vi "I-O Test.vi"() -> ()   [LabVIEW 2016]
uses:
  Classes/Controller/I-O/I-O.lvclass
  Classes/Controller/Controller.lvclass
panel:
  in  "secondary valve":bool
  in  "primary valve":bool
  out "Compression":bool=TRUE
  in  "Region Index":i32=1
  in  "Position Index":i32
  in  "Write":bool
  out "Read":bool
  in  "Stop":bool
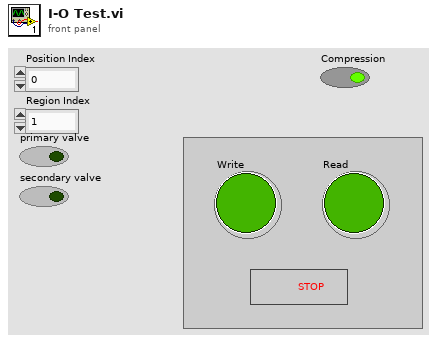
[diagram p1: front panel]
types:
  T1 = typedef "Controller.lvclass/Controllers.ctl" = cluster{"I-O.lvclass":refnum<class "I-O.lvclass">, "Motion.lvclass":refnum<class "Motion.lvclass">, "Dispenser.lvclass":refnum<class "Dispenser.lvclass">}
  T2 = typedef "I-O.lvclass/Pin Map.ctl" = cluster{"Region Valves":i32[], "Extra Valves":dbl[][], "Tool Primary Valve":i32, "Tool Secondary Valve":i32, "Region Sensors":i32[], "Extra Sensors":dbl[][], "Tool Primary Sensor":dbl, "Tool Secondary Sensor":dbl, "Compression Sensor":dbl, "5V":i32}
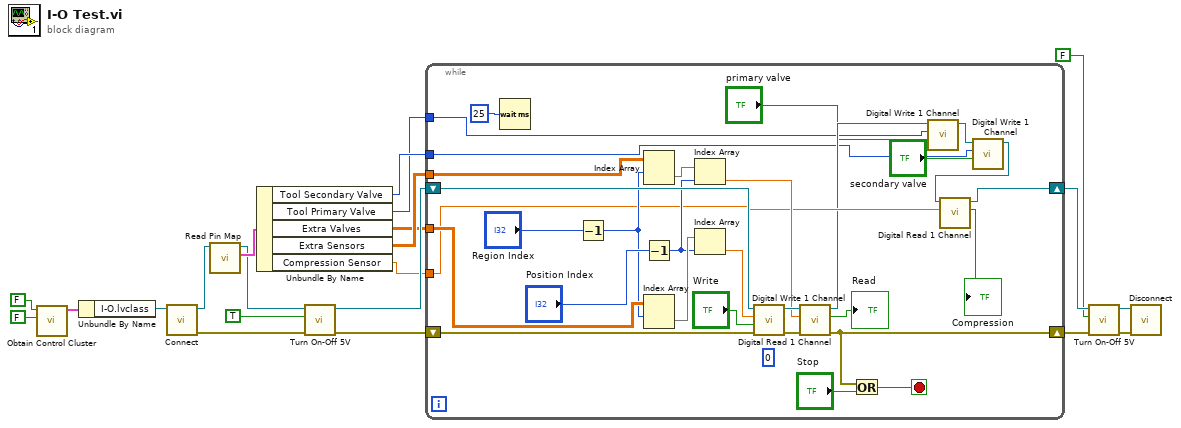
[diagram p0: block diagram]
diagram:
  n1 = call "Obtain Control Cluster.vi"("Dispense"=FALSE, "Motion"=FALSE) -> ("Control Out"=w5:T1)  [unwired: 9 in]
  n2 = Unbundle By Name(w5) -> ("I-O.lvclass"=w4:refnum<class "I-O.lvclass">)
  n3 = call-dynamic "Connect.vi"("Controller in"=w4) -> ("error out"=w12:errorcluster, "Controller out"=w14:refnum<class "I-O.lvclass">)  [unwired: 9 in]
  n4 = call-dynamic "Read Pin Map.vi"("I-O in"=w14) -> ("Pin Map"=w16:T2, "I-O out"=w15:refnum<class "I-O.lvclass">)  [unwired: 8 in, 1 out]
  n5 = Unbundle By Name(w16) -> ("Tool Secondary Valve"=w2:i32, "Tool Primary Valve"=w1:i32, "Extra Valves"=w8:dbl[][], "Extra Sensors"=w13:dbl[][], "Compression Sensor"=w3:dbl)
  n6 = call-dynamic "Turn On-Off 5V.vi"("error in (no error)"=w12, "Value"=TRUE, "I-O in"=w15) -> ("error out"=w11:errorcluster, "I-O out"=w21:refnum<class "I-O.lvclass">)  [unwired: 7 in]
  n7 = while {
    shift-right: [w29] -> w18
    shift-left: w21 -> [w50]
    tunnel: w13 -> [w37]
    shift-right: [w44] -> w10
    shift-left: w11 -> [w46]
    tunnel: w8 -> [w38]
    tunnel: w3 -> [w31]
    tunnel: w2 -> [w25]
    tunnel: w1 -> [w27]
    stop <- w42 stop-if-true
    (unwired) 0 ("disabled index (row)")
    n8 = Wait (ms)(milliseconds to wait=u32 25) -> ()  [unwired: 1 out]
    n9 = Decrement(x="Region Index") -> (x-1=w32:i32)
    n10 = Index Array(array=w37, index (row)=w32) -> (element=w34:dbl[])  [unwired: 1 in]
    n11 = Decrement(x="Position Index") -> (x-1=w33:i32)
    n12 = Index Array(array=w38, index (row)=w32) -> (element=w39:dbl[])  [unwired: 1 in]
    n13 = Index Array(array=w34, index=w33) -> (element=w40:dbl)
    n14 = Index Array(array=w39, index=w33) -> (element=w41:dbl)
    n15 = call-dynamic "Digital Write 1 Channel.vi"("error constant"=w46, "Value"="Write", "Channel"=w41, "I-O.lvclass"=w50) -> ("error IO"=w45:errorcluster, "I-O.lvclass 2"=w49:refnum<class "I-O.lvclass">)  [unwired: 6 in]
    n16 = call-dynamic "Digital Read 1 Channel.vi"("error in (no error)"=w45, "Read"=w40, "I-O in"=w49) -> ("error out"=w44:errorcluster, "Value"=→"Read":bool, "I-O out"=w28:refnum<class "I-O.lvclass">)  [unwired: 6 in]
    n17 = Or(x=w44, y="Stop") -> (x .or. y?=w42:bool)
    n18 = call-dynamic "Digital Write 1 Channel.vi"("Value"="primary valve", "Channel"=w27, "I-O.lvclass"=w28) -> ("I-O.lvclass 2"=w26:refnum<class "I-O.lvclass">)  [unwired: 7 in, 1 out]
    n19 = call-dynamic "Digital Write 1 Channel.vi"("Value"="secondary valve", "Channel"=w25, "I-O.lvclass"=w26) -> ("I-O.lvclass 2"=w22:refnum<class "I-O.lvclass">)  [unwired: 7 in, 1 out]
    n20 = call-dynamic "Digital Read 1 Channel.vi"("Read"=w31, "I-O in"=w22) -> ("Value"=→"Compression":bool, "I-O out"=w29:refnum<class "I-O.lvclass">)  [unwired: 7 in, 1 out]
  }
  n21 = call-dynamic "Turn On-Off 5V.vi"("error in (no error)"=w10, "Value"=FALSE, "I-O in"=w18) -> ("error out"=w9:errorcluster, "I-O out"=w19:refnum<class "I-O.lvclass">)  [unwired: 7 in]
  n22 = call-dynamic "Disconnect.vi"("error in (no error)"=w9, "I-O in"=w19) -> ()  [unwired: 8 in, 1 out]
